vi "Browse for XNET Database.vi"(8 "error in (no error)":errorcluster) -> (0 "error out":errorcluster, 1 "J1939 Monitor Settings":T1 {"Name" format="%.0x"}, 2 "Cancel Out":bool, 3 "J1939 XNET Settings":T2 {"Termination" items=["Off", "On"]})   [LabVIEW 2023, in "J1939 Addon System Explorer.lvlib"]
uses:
  J1939 Addon System Explorer.lvlib
  Addon Shared/Types/XNET Settings.ctl
  Addon Shared/Types/Monitor Settings.ctl
  <resource>/objmgr/xnet.rc
  Addon Shared/J1939 Addon Shared.lvlib
panel:
  in  "Name":u64=1 format="%.0x"
  in  "Address":u8 format="%.0x"
  in  "Baud rate [Bd]":u32=500000
  in  "Select CAN Cluster":u16(ring) items=["j1939.Cluster"]
  in  "Cancel":bool
  in  "Select":bool
  in  "XNET Database":refnum<k21>
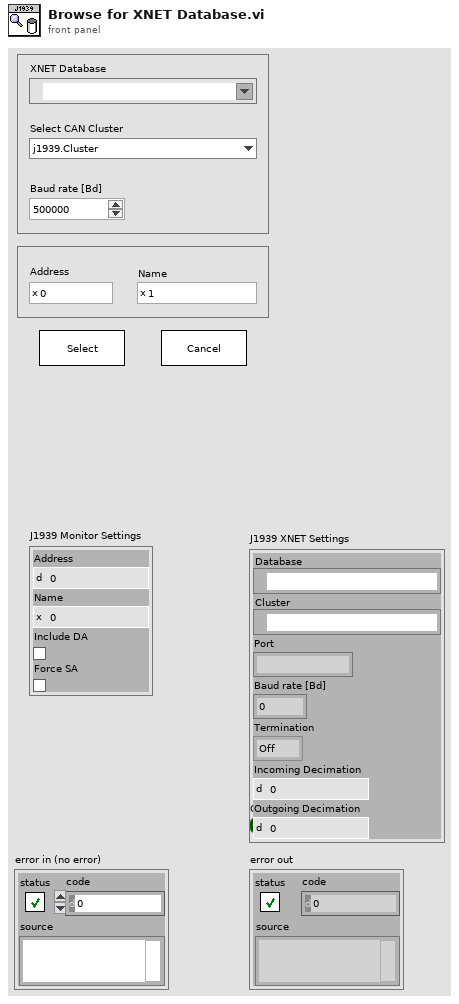
[diagram p1: front panel]
types:
  T1 = typedef "J1939 Addon Shared.lvlib/Monitor Settings.ctl" = cluster{"Address":u8, "Name":u64, "Include DA":bool, "Force SA":bool}
  T2 = typedef "J1939 Addon Shared.lvlib/XNET Settings.ctl" = cluster{"Database":refnum<k21>, "Cluster":refnum<k21>, "Port":string, "Baud rate [Bd]":u32, "Termination":u32, "Incoming Decimation":u32, "Outgoing Decimation":u32}
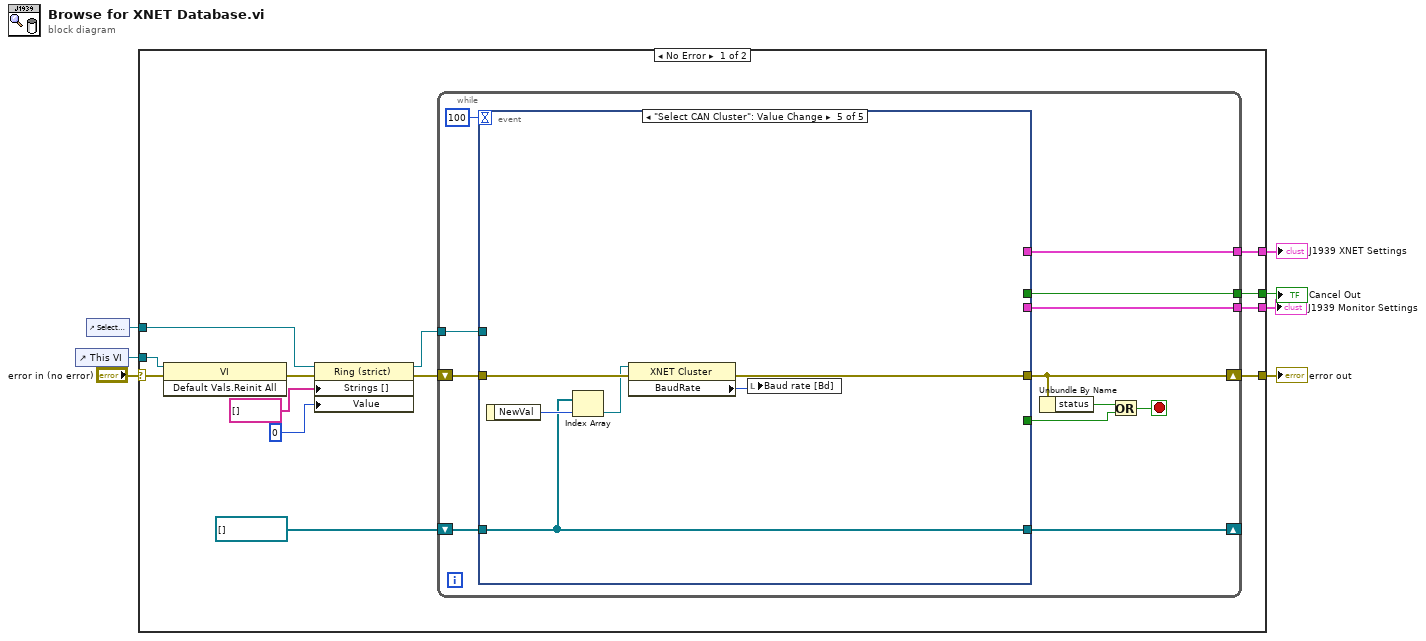
[diagram p0: block diagram]
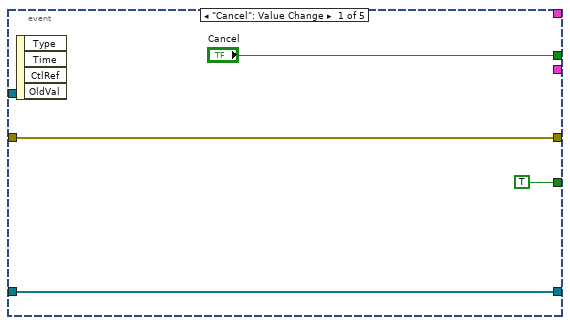
[diagram p2: hidden frame]
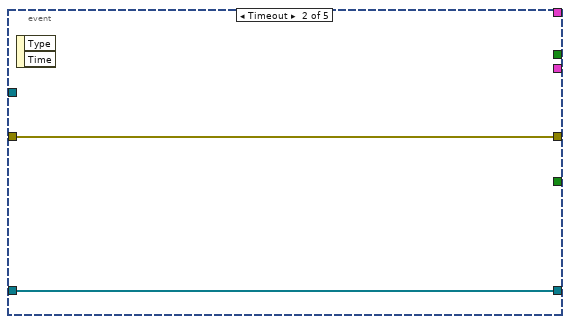
[diagram p3: hidden frame]
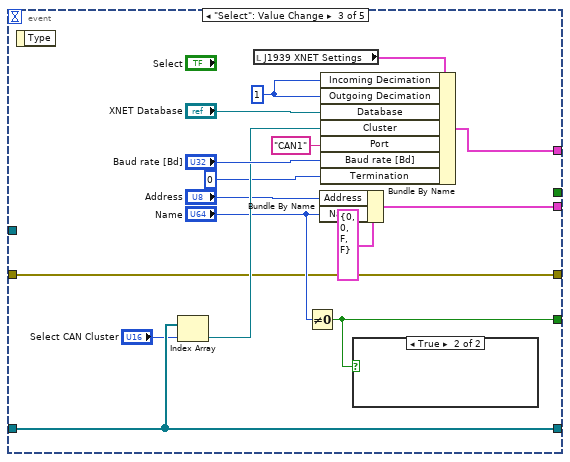
[diagram p4: hidden frame]
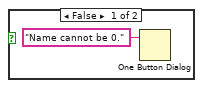
[diagram p5: hidden frame]
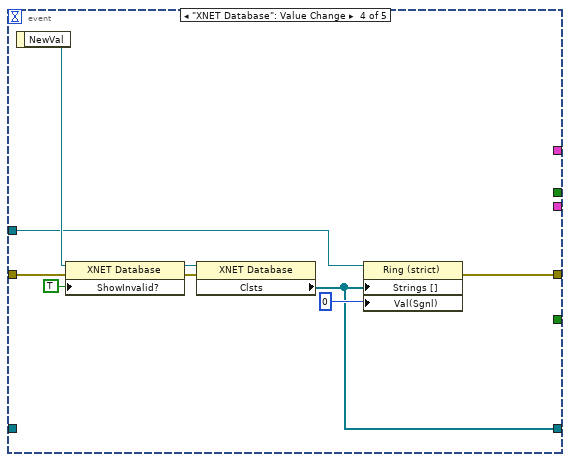
[diagram p6: hidden frame]
diagram:
  n1 = control-ref of="This VI"() -> (w4:refnum<vi>)
  n2 = control-ref of="Select CAN Cluster"() -> (w2:refnum<vi>)
  n3 = case shown="No Error" "error in (no error)" {
    selector: "error in (no error)" -> [w19 w71]
    tunnel: [w17 w71] -> w6
    tunnel: [w20 _] -> w5
    tunnel: w4 -> [w18 _]
    tunnel: [w15 _] -> w3
    tunnel: w2 -> [w14 _]
    tunnel: [w8 _] -> w1
    frame No Error {
      n4 = invoke class="VI" method="Default Vals.Reinit All"(reference=w18, error in=w19) -> (error out=w13:errorcluster)  [unwired: 1 in, 2 out]
      n5 = property on="Property Node" class="Ring (strict)"(reference=w14, error in=w13, "Strings []"=string[] [], "Value"=u16 0) -> (reference out=w12:refnum<vi>, error out=w11:errorcluster)
      n6 = while {
        tunnel: [w32] -> w20
        shift-right: [w30] -> _
        shift-left: refnum<k21>[] [] ("Clsts") -> [w29]
        shift-right: [w26] -> w17
        shift-left: w11 -> [w31]
        tunnel: [w28] -> w15
        tunnel: w12 -> [w22]
        tunnel: [w21] -> w8
        stop <- w23 stop-if-true
        n7 = event shown="[4] \"Select CAN Cluster\": Value Change" {
          selector: _ -> [_ _ _ _ _]
          dyn-events: _ -> [_ _ _ _ _]
          timeout: 100 -> [_ _ _ _ _]
          tunnel: ["Cancel" _ _ _ _] -> w32
          tunnel: w31 -> [w34 w38 w40 w61 w69]
          tunnel: [w35 w37 w51 w58 w65] -> w30
          tunnel: w29 -> [w35 w37 w51 _ w65]
          tunnel: [w34 w38 w40 w56 w68] -> w26
          tunnel: [_ _ w48 _ _] -> w28
          tunnel: [TRUE _ w41 _ _] -> w24
          tunnel: w22 -> [_ _ _ w57 _]
          tunnel: [_ _ w44 _ _] -> w21
          event "Cancel": Value Change {
            n8 = event-data() -> ()  [unwired: 1 in, 4 out]
          }
          event Timeout {
            n9 = event-data() -> ()  [unwired: 1 in, 2 out]
          }
          event "Select": Value Change {
            w43 = u32 1 ("Outcoming Rate")
            n10 = event-data() -> ()  [unwired: 1 in, 1 out]
            n11 = Index Array(array=w51, index="Select CAN Cluster") -> (element=w49:refnum<k21>)
            n12 = local read "J1939 XNET Settings"() -> (w52:T2)
            n13 = Not Equal To 0?(x="Name") -> (x != 0?=w41:bool)
            n14 = Bundle By Name(cluster=T1 {"Address"=0, "Name"=0, "Include DA"=FALSE, "Force SA"=FALSE} ("J1939 Monitor Settings"), "Address"="Address", "Name"="Name") -> (w44:T1)
            n15 = Bundle By Name(cluster=w52, "Incoming Decimation"=w43, "Outgoing Decimation"=w43, "Database"="XNET Database", "Cluster"=w49, "Port"="CAN1", "Baud rate [Bd]"="Baud rate [Bd]", "Termination"=u32 0) -> (w48:T2)
            n16 = case shown="True" w41 {
              frame False {
                n17 = One Button Dialog(message="Name cannot be 0.") -> ()  [unwired: 1 in, 1 out]
              }
              frame True {
              }
            }
          }
          event "XNET Database": Value Change {
            n18 = event-data() -> ("NewVal"=w60:refnum<k21>)  [unwired: 1 in]
            n19 = property class="XNET Database"(reference=w60, error in=w61, "ShowInvalid?"=TRUE ("Show Invalid From Open?")) -> (reference out=w64:refnum<k21>, error out=w63:errorcluster)
            n20 = property class="XNET Database"(reference=w64, error in=w63) -> ("Clsts"=w58:refnum<k21>[])  [unwired: 2 out]
            n21 = property on="Property Node" class="Ring (strict)"(reference=w57, "Strings []"=w58, "Val(Sgnl)"=u16 0 ("Value (Signaling)")) -> (error out=w56:errorcluster)  [unwired: 1 in, 1 out]
          }
          event "Select CAN Cluster": Value Change {
            n22 = event-data() -> ("NewVal"=w67:u16)  [unwired: 1 in]
            n23 = Index Array(array=w65, index=w67) -> (element=w66:refnum<k21>)
            n24 = property class="XNET Cluster"(reference=w66, error in=w69) -> (error out=w68:errorcluster, "BaudRate"=w70:u32)  [unwired: 1 out]
            n25 = local write "Baud rate [Bd]"(w70) -> ()
          }
        }
        n26 = Unbundle By Name(w26) -> ("status"=w25:bool)
        n27 = Or(x=w25, y=w24) -> (x .or. y?=w23:bool)
      }
    }
    frame Error {
    }
  }
  "error out" <- w6
  "Cancel Out" <- w5
  "J1939 XNET Settings" <- w3
  "J1939 Monitor Settings" <- w1
